vi "testDFA_2.vi"(8 "error in (no error)":errorcluster, 11 "TestCase in":refnum<class "DFA Tester.lvclass">) -> (0 "error out":errorcluster, 3 "TestCase out":refnum<class "DFA Tester.lvclass">)   [LabVIEW 2016, in "Assert API Components.lvlib" / "Log Assert Core.lvlib" / "DFA Tester.lvclass"]
uses:
  DFA Tester.lvclass
  Core/Assert API Components/Message Data.ctl
  Core/Assert API Components/Failure Actions.ctl
  Core/Assert API Components/VI References.ctl
  Core/Assert API Components/Log Assert Core Components/Event Transmission/Failure Action Change Event Reference.ctl
  DFA Tester.lvclass/DFA Tester.ctl
  <vilib>/addons/_JKI Toolkits/VI Tester/TestCase.llb/TestCase.lvclass
  Core/Assert API Components/Log Assert Core Components/Log Assert Core.lvlib
  Core/Assert API Components/Assert API Components.lvlib
  C:/Program Files (x86)/National Instruments/LabVIEW 2016/vi.lib/addons/_JKI Toolkits/VI Tester/TestCase.llb/TestCase.lvclass
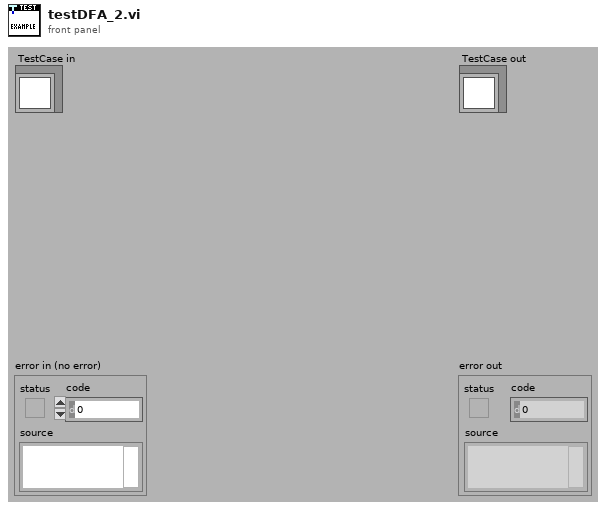
[diagram p1: front panel]
types:
  T1 = typedef "Assert API Components.lvlib/Message Data.ctl" = cluster{"Data Value":variant, "Last Update":timestamp, "Comment":string, "Evaluation String":string, "Status":bool, "Assert Name":string, "Failure Action":T2, "Assert VI Name":string, "Calling VI Name":string, "Assert VI UID":i32, "Top Level VI Name":string, "VI References":T3, "Assert Build Timestamp":timestamp, "Assert Builder User Name":string, "Data Type":string, "IP Address":string}
  T2 = typedef "Assert API Components.lvlib/Failure Actions.ctl" = enum16{"None", "Log To File", "Pause Execution", "Abort Execution"}
  T3 = typedef "Assert API Components.lvlib/VI References.ctl" = cluster{"Calling VI Ref":refnum<vi>, "Assert VI Ref":refnum<vi>}
  T4 = typedef "Assert API Components.lvlib/Log Assert Core.lvlib/Failure Action Change Event Reference.ctl" = cluster{"Failure Action Change Event":refnum<user-event>, "Event Registration Refnum":refnum<event-registration>}
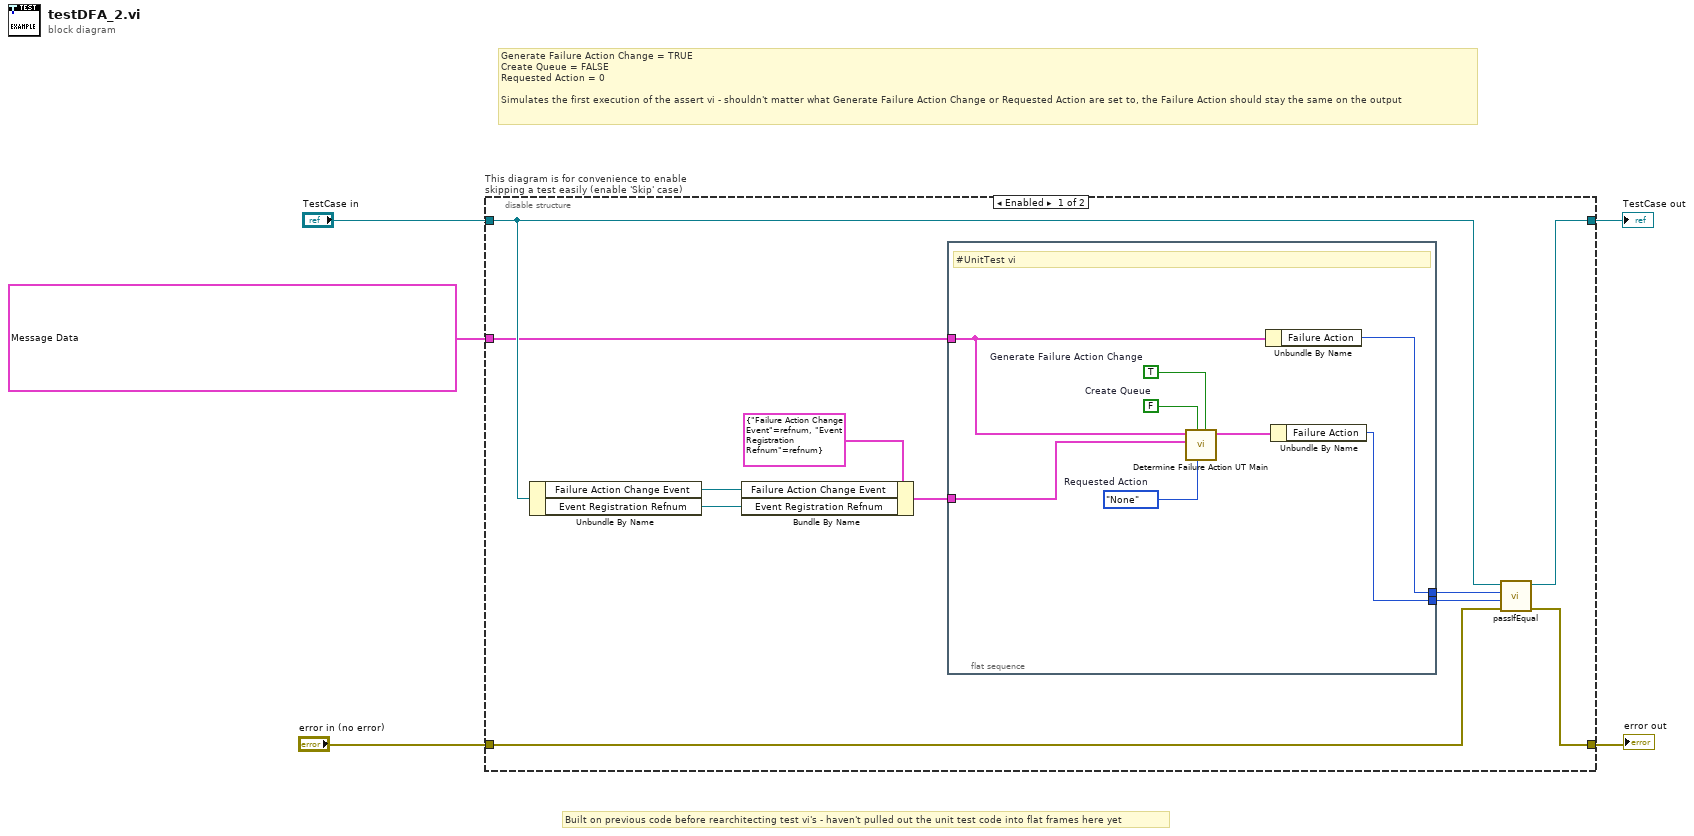
[diagram p0: block diagram]
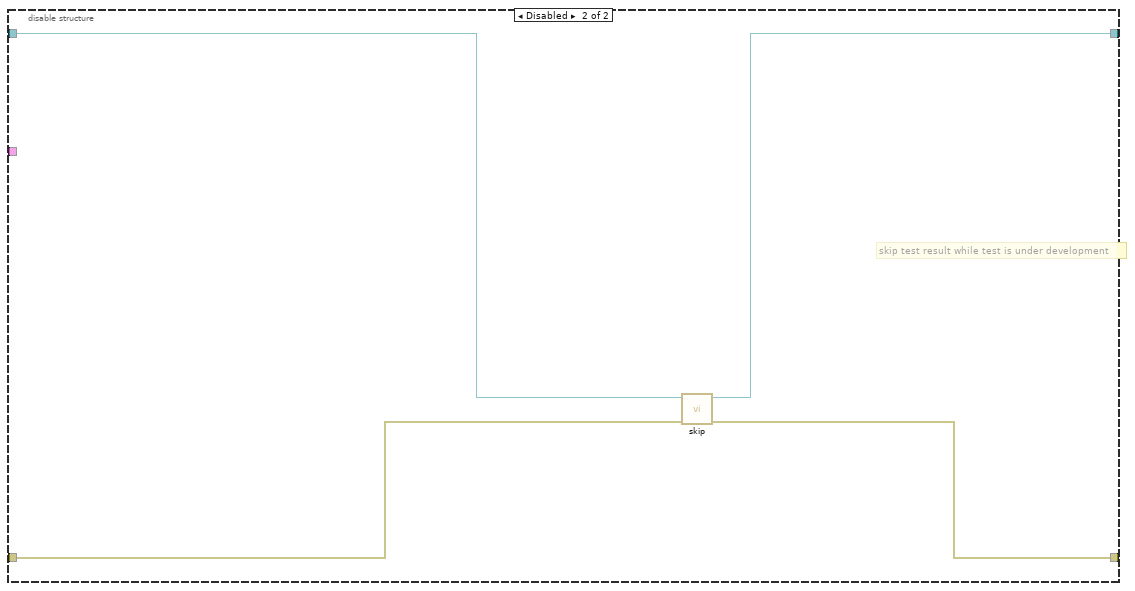
[diagram p2: hidden frame]
diagram:
  # "Built on previous code before rearchitecting test vi's - haven't pulled out the unit test code into flat frames here yet"
  # "Generate Failure Action Change = TRUE\nCreate Queue = FALSE\nRequested Action = 0\n\nSimulates the first execution of the assert vi - shouldn't matter what Generate Failure Action Change or Requested Action are set to, the Failure Action should stay the same on the output"
  n1 = disable-structure "This diagram is for convenience to enable skipping a test easily (enable 'Skip' case)" shown="Enabled" {
    disable-tunnel: "TestCase in" -> [w11 w28]
    disable-tunnel: [w16 w26] -> w2
    disable-tunnel: [w15 w27] -> w4
    disable-tunnel: "error in (no error)" -> [w14 w25]
    disable-tunnel: T1 {"Data Value"=variant, "Last Update"=timestamp(0 s since 1904-01-01), "Comment"="", "Evaluation String"="", "Status"=FALSE, "Assert Name"="", "Failure Action"=enum."None", "Assert VI Name"="", "Calling VI Name"="", "Assert VI UID"=0, "Top Level VI Name"="", "VI References"={"Calling VI Ref"=refnum, "Assert VI Ref"=refnum}, "Assert Build Timestamp"=timestamp(0 s since 1904-01-01), "Assert Builder User Name"="", "Data Type"="", "IP Address"=""} ("Assert Message in") -> [w8 _]
    frame Enabled {
      n2 = Unbundle By Name(w11) -> ("Failure Action Change Event"=w10:refnum<user-event>, "Event Registration Refnum"=w9:refnum<event-registration>)
      n3 = Bundle By Name(cluster=T4 {"Failure Action Change Event"=refnum, "Event Registration Refnum"=refnum} ("Failure Action Change Event References in"), "Failure Action Change Event"=w10, "Event Registration Refnum"=w9) -> (w12:T4)
      n4 = flat-sequence {
        tunnel: [w19] -> w7
        tunnel: [w18] -> w6
        tunnel: w12 -> [w22]
        tunnel: w8 -> [w21]
        frame #0 {
          w17 = TRUE  # Generate Failure Action Change
          w23 = Failure_Actions."None"  # Requested Action
          w24 = FALSE  # Create Queue
          # "#UnitTest vi"
          n5 = call "Determine Failure Action UT Main.vi"("Generate Failure Action Change"=w17, "Requested Action"=w23, "Create Queue"=w24, "Failure Action Change Event References in"=w22, "Assert Message in"=w21) -> ("Assert Message out"=w20:T1)  [unwired: 5 in, 1 out]
          n6 = Unbundle By Name(w21) -> ("Failure Action"=w19:T2)
          n7 = Unbundle By Name(w20) -> ("Failure Action"=w18:T2)
        }
      }
      n8 = call-dynamic "passIfEqual.vi"("error in (no error)"=w14, "y"=w6, "x"=w7, "TestCase in"=w11) -> ("error out"=w15:errorcluster, "TestCase out"=w16:refnum<class "DFA Tester.lvclass">)  [unwired: 6 in]
    }
    frame Disabled {
      # "skip test result while test is under development"
      n9 = call <vilib>:"skip.vi"("error in (no error)"=w25, "TestCase in"=w28) -> ("error out"=w27:errorcluster, "TestCase out"=w26:refnum<class "DFA Tester.lvclass">)  [unwired: 8 in]
    }
  }
  "error out" <- w4
  "TestCase out" <- w2
